vi "FTW-Actor-GetInstanceReference.vi"(11 "error in":errorcluster) -> (4 "Actor Refnum":refnum<vi>, 15 "error out":errorcluster)   [LabVIEW 2015, in "FTW-ActorInstance.lvclass"]
doc: "This VI is intended to only be used by actors in special cases where the actor reference cannot be passed down by the actor and only works with dynamic dispatch actors"
uses:
  FTW-ActorInstance.lvclass
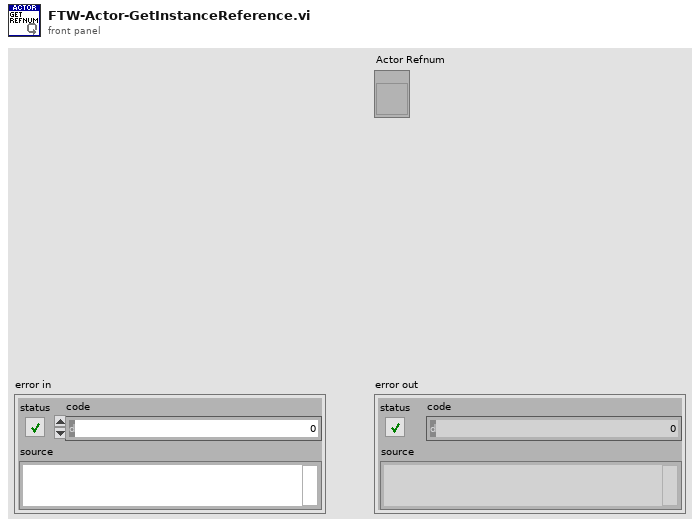
[diagram p1: front panel]
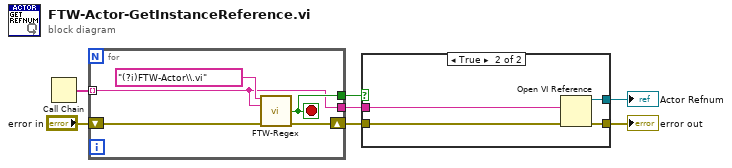
[diagram p0: block diagram]
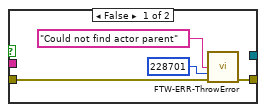
[diagram p2: hidden frame]
diagram:
  n1 = Call Chain() -> (call chain=w7:string[])
  n2 = for {
    tunnel: w7 -> [w10] mode=indexing
    tunnel: [w11] -> w5
    tunnel: [w10] -> w6
    shift-right: [w8] -> w3
    shift-left: "error in" -> [w9]
    stop <- w11 stop-if-true
    n3 = call "FTW-Regex.vi"("Regular Expression"="(?i)FTW-Actor\\.vi" ("regular expression"), "Input String"=w10, "error in"=w9) -> ("Match Found?"=w11:bool, "error out"=w8:errorcluster)  [unwired: 8 in, 3 out]
  }
  n4 = case shown="True" w5 {
    tunnel: w6 -> [_ w20]
    tunnel: w3 -> [w16 w19]
    tunnel: [w15 w18] -> w2
    tunnel: [_ w17] -> w1
    frame False {
      n5 = call "FTW-ERR-ThrowError.vi"("Error Message"="Could not find actor parent", "Error Code"=228701, "error in"=w16) -> ("error out"=w15:errorcluster)  [unwired: 12 in]
    }
    frame True {
      n6 = Open VI Reference(vi path=w20, error in (no error)=w19) -> (vi reference=w17:refnum<vi>, error out=w18:errorcluster)  [unwired: 4 in]
    }
  }
  "Actor Refnum" <- w1
  "error out" <- w2
